vi "全局流量数据小时.vi"() -> ()   [LabVIEW 2016]
panel:
  in  "累积流量":string[][](array[string])
  in  "瞬时流量":string[][](array[string])
  in  "流速":string[][](array[string])
  in  "水位":string[][](array[string])
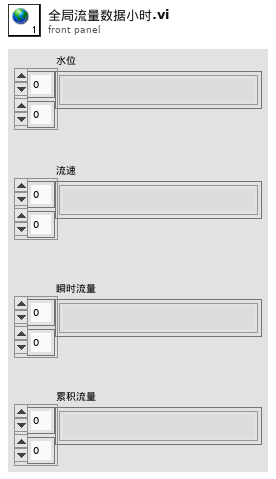
[diagram p1: front panel]
diagram:
